vi "Core Read DAQ FIFO.vi"(7 "Release Lock":bool=TRUE, 8 "error in (no error)":errorcluster, 9 "Timeout (ms)":i32=100, 10 "DAQ In":T1[](array[typedef]), 11 "CIFTag in":refnum<class "CIF_NIChn_Fifo_DAQ.lvclass">) -> (0 "error out":errorcluster, 1 "timed out?":bool, 2 "DAQ Out":T1[](array[typedef]), 3 "CIFTag out":refnum<class "CIF_NIChn_Fifo_DAQ.lvclass">, 4 "Header":T2)   [LabVIEW 2021, in "CIF_NIChn_Fifo_DAQ.lvclass"]
uses:
  CIF_NIChn_Fifo_DAQ.lvclass
  D:/dev/Packages/Channel_Manager/src/CIFChannels/CIFChannels.lvclass
  D:/dev/Packages/Channel_Manager/src/CIF_NIChn/NIChn/CIF_NIChn.lvclass
  ChannelCommon/typedef/FIFO Header.ctl
  ChannelCommon/typedef/Datatype Waveform.ctl
  CIFChannels/CIFChannels.lvclass/CIFChannels.ctl
  NIChn/CIF_NIChn.lvclass/CIF_NIChn.ctl
  CIF_NIChn_Fifo_DAQ.lvclass/CIF_NIChn_Fifo_DAQ.ctl
  ChannelCommon/CIFFIFO/CIFfifo.lvclass/CIFfifo.ctl
  NIChn/Accessors/Read CIF Channel.vi
  NIChn/SubVIs/Check Disconnect.vi
  <vilib>/CIFChannels/Top Level/Read Variable Length U8 Array.vi
  NIChn/Accessors/Write CIF Channel.vi
  Unflatten.vi
  CIFChannels/Accessors/Read Channel State.vi
  CIFChannels/Accessors/Read Direction.vi
  CIFChannels/Accessors/Write Channel State.vi
  CIFChannels/Accessors/Read Tag Disconnect Behavior.vi
  <vilib>/CIFChannels/Top Level/Read Variable Length U8 Array.vi/81056090-23cf-424a-a716-29db01c8ef1b.vi
  <vilib>/CIFChannels/Top Level/Read Variable Length U8 Array.vi/6610cd62-0a6d-4591-8fd4-6453482a4bc1.vi
  <vilib>/CIFChannels/Top Level/Read Variable Length U8 Array.vi/93d598b0-524b-4f76-9570-a74a86ef2c6f.vi
  ChannelCommon/CIFFIFO/Accessors/Write Timeout.vi
  ChannelCommon/CIFFIFO/Flatten/DVR Unflatten.vi
  ChannelCommon/CIFFIFO/Accessors/Write Header.vi
  <vilib>/CIFChannels/Top Level/Read Variable Length U8 Array.vi/81056090-23cf-424a-a716-29db01c8ef1b.vi/4bc1c15b-36ab-481f-b8dd-c64075ce723a.vi
  <vilib>/CIFChannels/Top Level/Read Variable Length U8 Array.vi/81056090-23cf-424a-a716-29db01c8ef1b.vi/d83cb72b-7713-41fc-a3d1-682de79cf574.vi
  <vilib>/CIFChannels/SubVIs/Get dll Path.vi
  <vilib>/CIFChannels/Top Level/Read Variable Length U8 Array.vi/6610cd62-0a6d-4591-8fd4-6453482a4bc1.vi/c28b0ead-42ad-4072-80a2-aca7f2bd7ce3.vi
  <vilib>/CIFChannels/Top Level/Read Variable Length U8 Array.vi/93d598b0-524b-4f76-9570-a74a86ef2c6f.vi/4bc1c15b-36ab-481f-b8dd-c64075ce723a.vi
  <vilib>/CIFChannels/Top Level/Read Variable Length U8 Array.vi/93d598b0-524b-4f76-9570-a74a86ef2c6f.vi/d83cb72b-7713-41fc-a3d1-682de79cf574.vi
  ChannelCommon/Utilities/Unflatten Header.vi
  ChannelCommon/Utilities/Add Error.vi
  <vilib>/CIF Foundation/CIF Utilities/DataTypes/Unflatten U64.vi
  <vilib>/CIF Foundation/CIF Utilities/DataTypes/Unflatten I64.vi
  <vilib>/CIF Foundation/CIF Utilities/Errors/Append Error Location.vi
  NIChn/CIF_NIChn.lvclass
  ChannelCommon/ChannelCommon.lvlib
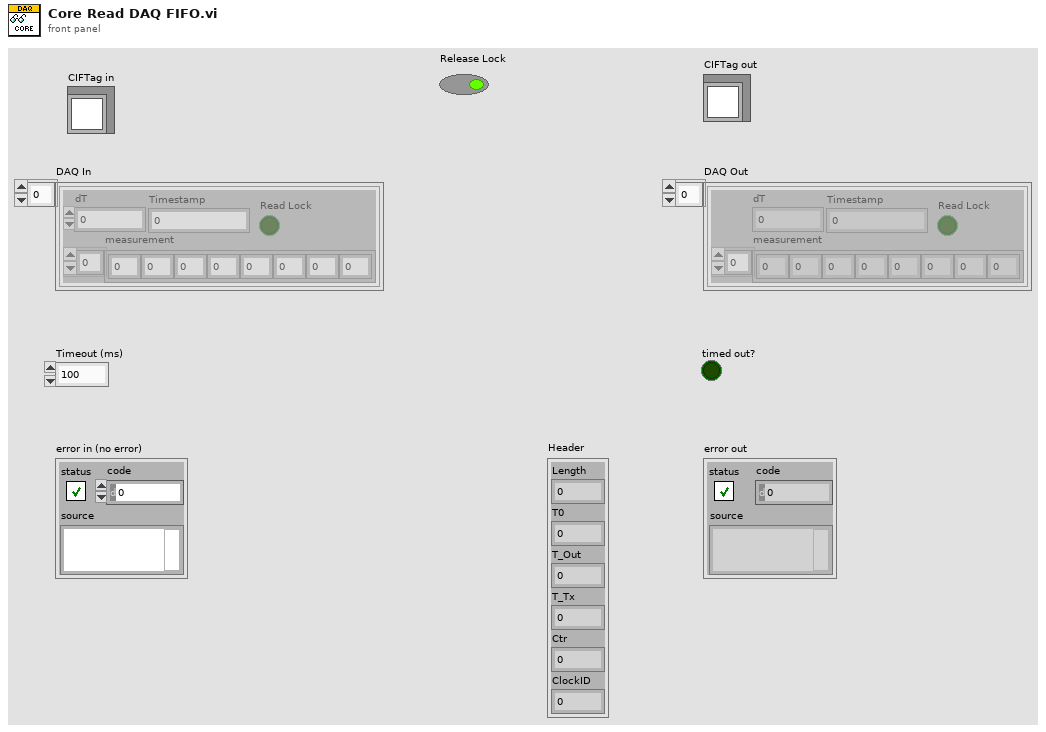
[diagram p1: front panel]
types:
  T1 = typedef "ChannelCommon.lvlib/Datatype Waveform.ctl" = cluster{"measurement":dbl[], "dT":dbl, "Timestamp":u64, "Read Lock":bool}
  T2 = typedef "ChannelCommon.lvlib/FIFO Header.ctl" = cluster{"Length":u64, "T0":i64, "T_Out":i64, "T_Tx":i64, "Ctr":u64, "ClockID":u8}
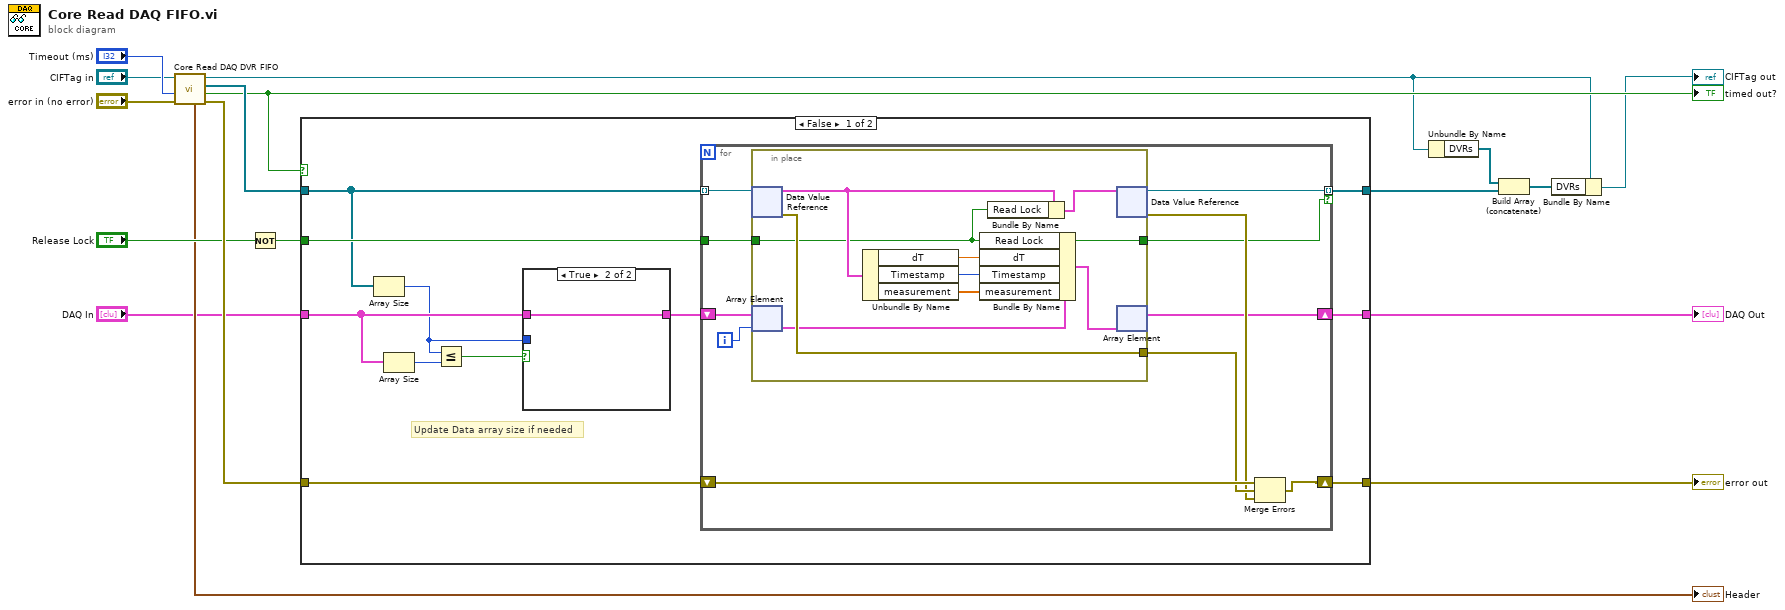
[diagram p0: block diagram]
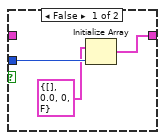
[diagram p2: hidden frame]
diagram:
  n1 = call "Core Read DAQ DVR FIFO.vi"("error in (no error)"="error in (no error)", "Timeout (ms)"="Timeout (ms)", "CIFTag in"="CIFTag in") -> ("error out"=w17:errorcluster, "timed out?"=w12:bool, "Data Out"=w16:refnum<data-value>[], "CIFTag out"=w8:refnum<class "CIF_NIChn_Fifo_DAQ.lvclass">, "Header"=→"Header":T2)  [unwired: 4 in]
  "timed out?" <- w12
  n2 = Not(x="Release Lock") -> (.not. x?=w14:bool)
  n3 = case shown="False" w12 {
    tunnel: w17 -> [w28 w54]
    tunnel: w16 -> [w19 _]
    tunnel: [w25 w54] -> w13
    tunnel: "DAQ In" -> [w21 w53]
    tunnel: w14 -> [w27 _]
    tunnel: [w26 w53] -> w3
    tunnel: [w24 _] -> w6
    frame False {
      # "Update Data array size if needed"
      n4 = Array Size(array=w19) -> (size(s)=w18:i32)
      n5 = Array Size(array=w21) -> (size(s)=w22:i32)
      n6 = Less Or Equal?(x=w18, y=w22) -> (x <= y?=w23:bool)
      n7 = case shown="True" w23 {
        tunnel: w21 -> [_ w32]
        tunnel: [w29 w32] -> w20
        tunnel: w18 -> [w31 _]
        frame False {
          n8 = Initialize Array(T1 {"measurement"=[], "dT"=0.0, "Timestamp"=0, "Read Lock"=FALSE} ("Waveform Datatype"), w31) -> (w29:T1[])
        }
        frame True {
        }
      }
      n9 = for {
        tunnel: w19 -> [w43] mode=indexing
        shift-right: [w39] -> w25
        shift-left: w28 -> [w42]
        shift-right: [w34] -> w26
        shift-left: w20 -> [w35]
        tunnel: w27 -> [w38]
        tunnel: [w37] -> w24 mode=indexing if=w36
        i -> [w33]
        n10 = in-place {
          in-place-border: [w52] -> w41
          in-place-border: w38 -> [w49]
          in-place-border: [w49] -> w36
          n11 = in-place-dvr #1(w43) -> (w51:T1, w52:errorcluster)
          n12 = in-place-array #2(w35, w33) -> (w45:T1)
          n13 = Unbundle By Name(w51) -> ("dT"=w46:dbl, "Timestamp"=w47:u64, "measurement"=w48:dbl[])
          n14 = Bundle By Name(cluster=w45, "Read Lock"=w49, "dT"=w46, "Timestamp"=w47, "measurement"=w48) -> (w44:T1)
          n15 = Bundle By Name(cluster=w51, "Read Lock"=w49) -> (w50:T1)
          n16 = in-place-dvr #1(w50) -> (w37:refnum<data-value>, w40:errorcluster)
          n17 = in-place-array #2(w44) -> (w34:T1[])  [unwired: 1 out]
        }
        n18 = Merge Errors(w42, w41, w40) -> (w39:errorcluster)
      }
    }
    frame True {
    }
  }
  "error out" <- w13
  "DAQ Out" <- w3
  n19 = Unbundle By Name(w8) -> ("DVRs"=w7:refnum<data-value>[])
  n20 = Build Array (concatenate)(w7, w6) -> (w5:refnum<data-value>[])
  n21 = Bundle By Name(cluster=w8, "DVRs"=w5) -> (→"CIFTag out":refnum<class "CIF_NIChn_Fifo_DAQ.lvclass">)
